vi "AdvSigProc_Create.vi"(0 "reference in":refnum<class "AdvSigProc.lvclass">, 5 "error in (no error)":errorcluster, 6 "Time Data":refnum<class "GSwFormDSP.lvclass">, 7 "Application Name":string, 9 "State Queue":string[](array[string])) -> (14 "reference out":refnum<class "AdvSigProc.lvclass">, 19 "error out":errorcluster)   [LabVIEW 2022 SP3, in "AdvSigProc.lvclass"]
doc: "Constructor."
uses:
  AdvSigProc.lvclass
  C:/Program Files/National Instruments/LabVIEW 2022/vi.lib/addons/_AddQ/G#Object/G#Object.lvclass
  W:/projects/archives/23 Charette AI Group/SPWB/API/Generic Utilities_class/Generic Utilities.lvclass
  API/GSwFormDSP_class/GSwFormDSP.lvclass
  <vilib>/addons/_AddQ/G#Object/G#Object.lvclass
  API/Generic Utilities_class/Generic Utilities.lvclass
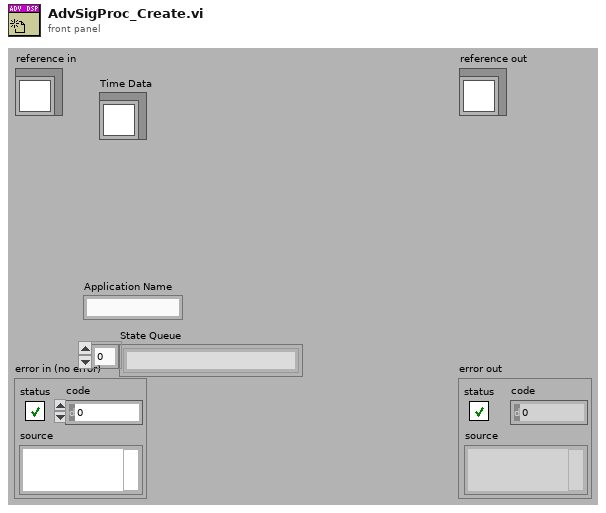
[diagram p1: front panel]
types:
  T1 = typedef "AdvSigProc.lvclass/ObjectAttributesRef.ctl" = refnum<data-value>
  T2 = typedef "AdvSigProc.lvclass/ObjectAttributes.ctl" = cluster{"Time Data":cluster{"New Time Data Obj?":bool, "GSwFormDSP":refnum<class "GSwFormDSP.lvclass">}, "LMS Parameters":T3}
  T3 = typedef "AdvSigProc.lvclass/LMS.ctl" = cluster{"adaptive filter Ref":refnum<k20>, "Filtered Signals":refnum<class "GSwFormDSP.lvclass">, "Filter Coefs":dbl[], "Input Parameters":T4, "Iteration Metrics":T5[]}
  T4 = typedef "AdvSigProc.lvclass/LMS Input Parameters.ctl" = cluster{"Type":enum16{"Normalized LMS", "LMS", "FIR Sign LMS", "FIR Fast Block LMS", "RLS", "QR - RLS"}, "Filter Class":enum16{"Noise Cancelling (BGN Ref)", "Noise Cancelling (Speech Ref)"}, "Filter Length":i32, "µ Parameters":cluster{"Type":enum16{"User Input", "Auto µ"}, "step size":dbl}, "Iterations":cluster{"Current":i32, "Maximum":i32}}
  T5 = typedef "AdvSigProc.lvclass/Iteration Metrics.ctl" = cluster{"Name":string, "Max":dbl, "Min":dbl, "Values History":dbl[]}
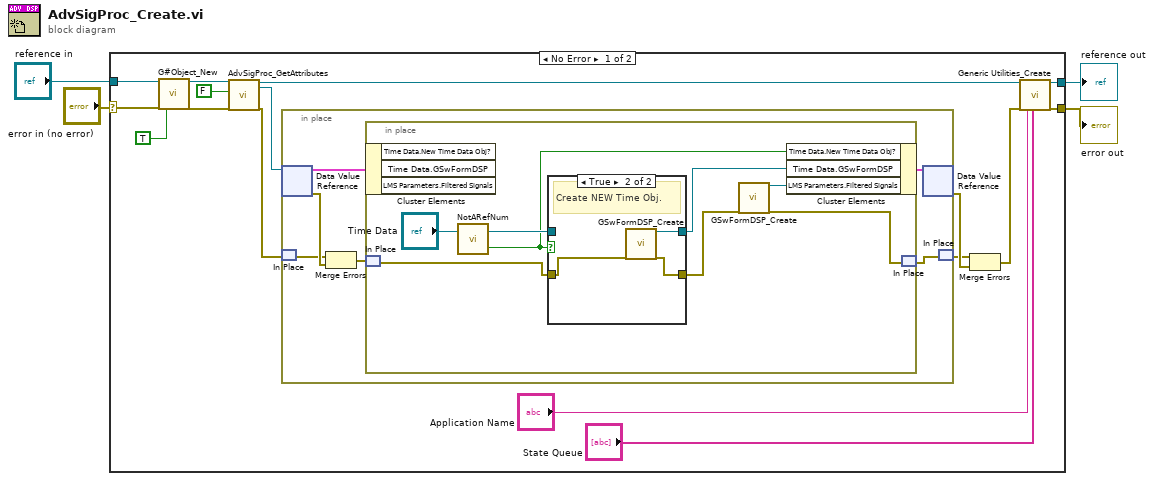
[diagram p0: block diagram]
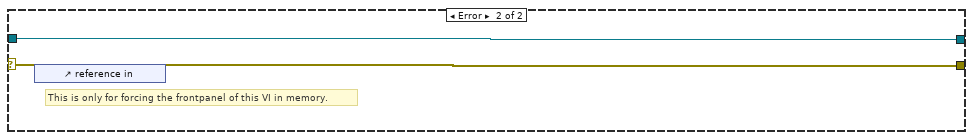
[diagram p3: hidden frame]
diagram:
  n1 = case shown="No Error" "error in (no error)" {
    selector: "error in (no error)" -> [w19 w41]
    tunnel: [w9 w41] -> w3
    tunnel: [w11 w40] -> w1
    tunnel: "reference in" -> [w20 w40]
    frame No Error {
      n2 = call <vilib>:"G#Object_New.vi"("reference in"=w20, "error in (no error)"=w19, "user counter (T)?"=TRUE ("User Counter")) -> ("reference out"=w14:refnum<class "AdvSigProc.lvclass">, "error out"=w13:errorcluster)  [unwired: 14 in, 1 out]
      n3 = call "AdvSigProc_GetAttributes.vi"("reference in"=w14, "return data? (T)"=FALSE ("return data"), "error in (no error)"=w13) -> ("reference out"=w12:refnum<class "AdvSigProc.lvclass">, "attributes ref"=w16:T1, "error out"=w8:errorcluster)  [unwired: 13 in, 1 out]
      n4 = in-place {
        n5 = in-place-dvr #1(w16) -> (w25:T2, w24:errorcluster)
        n6 = in-place-match #2(w8) -> (w23:errorcluster)
        n7 = Merge Errors(w23, w24) -> (w22:errorcluster)
        n8 = in-place {
          n9 = in-place-cluster #3(w25) -> ()  [unwired: 3 out]
          n10 = in-place-match #4(w22) -> (w30:errorcluster)
          n11 = call-dynamic "NotARefNum.vi"("reference in"="Time Data") -> ("not a refnum?"=w31:bool, "reference out"=w32:refnum<class "GSwFormDSP.lvclass">)  [unwired: 1 in]
          n12 = case shown="True" w31 {
            tunnel: [w36 w37] -> w34
            tunnel: w32 -> [w36 _]
            tunnel: w30 -> [w35 w39]
            tunnel: [w35 w38] -> w28
            frame False {
              # "Copy an existing reference."
            }
            frame True {
              # "Create NEW Time Obj."
              n13 = call "GSwFormDSP_Create.vi"("error in (no error)"=w39) -> ("reference out"=w37:refnum<class "GSwFormDSP.lvclass">, "error out"=w38:errorcluster)  [unwired: 17 in]
            }
          }
          n14 = call "GSwFormDSP_Create.vi"("error in (no error)"=w28) -> ("reference out"=w29:refnum<class "GSwFormDSP.lvclass">, "error out"=w27:errorcluster)  [unwired: 17 in]
          n15 = in-place-cluster #3("Time Data.New Time Data Obj?"=w31, "Time Data.GSwFormDSP"=w34, "LMS Parameters.Filtered Signals"=w29) -> (w26:T2)
          n16 = in-place-match #4(w27) -> (w21:errorcluster)
        }
        n17 = in-place-dvr #1(w26) -> (w17:errorcluster)  [unwired: 1 out]
        n18 = in-place-match #2(w21) -> (w7:errorcluster)
      }
      n19 = Merge Errors(w7, w17) -> (w10:errorcluster)
      n20 = call "Generic Utilities_Create.vi"("reference in"=w12, "error in (no error)"=w10, "Application Name"="Application Name", "State Queue"="State Queue") -> ("reference out"=w11:refnum<class "AdvSigProc.lvclass">, "error out"=w9:errorcluster)  [unwired: 14 in]
    }
    frame Error {
      # "This is only for forcing the frontpanel of this VI in memory."
      n21 = control-ref of="reference in"() -> ()  [unwired: 1 out]
    }
  }
  "error out" <- w3
  "reference out" <- w1
